vi "SaveScriptFile.vi"(9 "file name":string="scriptmain.py", 11 "text":string) -> (3 "source":string)   [LabVIEW 2019]
uses:
  System.Windows.Forms
panel:
  in  ".NET Refnum in 2":refnum<k24>
  out "source 2":string
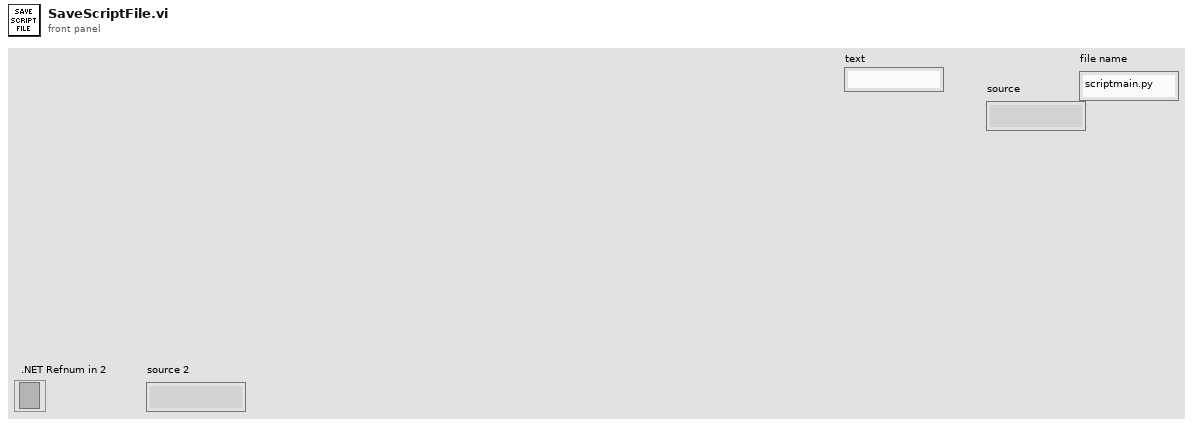
[diagram p1: front panel]
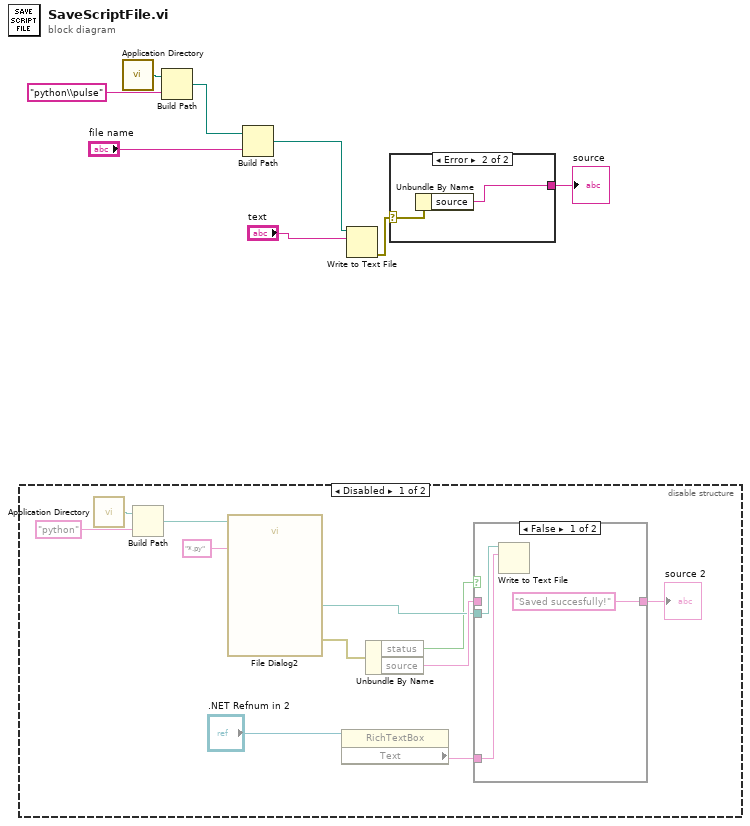
[diagram p0: block diagram]
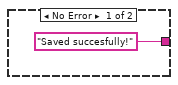
[diagram p4: hidden frame]
diagram:
  n1 = disable-structure shown="Disabled" {
    frame Disabled {
      n2 = call <vilib>:"Application Directory.vi"() -> ("Application Directory"=w9:path)
      n3 = Build Path(base path=w9, name or relative path="python") -> (appended path=w11:path)
      n4 = call "File Dialog2"("start path"=w11, "pattern (all files)"="*.py") -> ("selected path"=w15:path, "error out"=w13:errorcluster)  [unwired: 10 in, 2 out]
      n5 = property class="RichTextBox"(reference=".NET Refnum in 2") -> ("Text"=w17:string)  [unwired: 1 in, 2 out]
      n6 = Unbundle By Name(w13) -> ("status"=w14:bool, "source"=w18:string)
      n7 = case shown="False" w14 {
        tunnel: w15 -> [w22 _]
        tunnel: w17 -> [w21 _]
        tunnel: w18 -> [_ w23]
        tunnel: ["Saved succesfully!" ("source") w23] -> w19
        frame False {
          n8 = Write to Text File(file (use dialog)=w22, text=w21) -> ()  [unwired: 2 in, 3 out]
        }
        frame True {
        }
      }
      "source 2" <- w19
    }
    frame Enabled {
    }
  }
  n9 = call <vilib>:"Application Directory.vi"() -> ("Application Directory"=w6:path)
  n10 = Build Path(base path=w6, name or relative path="python\\pulse") -> (appended path=w4:path)
  n11 = Build Path(base path=w4, name or relative path="file name") -> (appended path=w2:path)
  n12 = Write to Text File(file (use dialog)=w2, text="text") -> (error out=w5:errorcluster)  [unwired: 2 in, 2 out]
  n13 = case shown="Error" w5 {
    selector: w5 -> [_ w26]
    tunnel: ["Saved succesfully!" ("source") w25] -> w8
    frame No Error {
    }
    frame Error {
      n14 = Unbundle By Name(w26) -> ("source"=w25:string)
    }
  }
  "source" <- w8
